vi "Write Target-FIFO 16ch.vi"(0 "16xIQ in":T1=[{"I"=0.0, "Q"=0.0, "overflow"=FALSE}, {"I"=0.0, "Q"=0.0, "overflow"=FALSE}, {"I"=0.0, "Q"=0.0, "overflow"=FALSE}, {"I"=0.0, "Q"=0.0, "overflow"=FALSE}, {"I"=0.0, "Q"=0.0, "overflow"=FALSE}, {"I"=0.0, "Q"=0.0, "overflow"=FALSE}, {"I"=0.0, "Q"=0.0, "overflow"=FALSE}, {"I"=0.0, "Q"=0.0, "overflow"=FALSE}, {"I"=0.0, "Q"=0.0, "overflow"=FALSE}, {"I"=0.0, "Q"=0.0, "overflow"=FALSE}, {"I"=0.0, "Q"=0.0, "overflow"=FALSE}, {"I"=0.0, "Q"=0.0, "overflow"=FALSE}, {"I"=0.0, "Q"=0.0, "overflow"=FALSE}, {"I"=0.0, "Q"=0.0, "overflow"=FALSE}, {"I"=0.0, "Q"=0.0, "overflow"=FALSE}, {"I"=0.0, "Q"=0.0, "overflow"=FALSE}], 7 "Ch select":i32, 9 "input valid":bool) -> (3 "DSP Overflow":bool, 10 "Timed Out?":bool)   [LabVIEW 2015, in "DDC_7976R_v1.lvlib"]
uses:
  DDC_7976R_v1.lvlib
  16xIQData.ctl
  <instrlib>/_niInstr/DSP/v1/Shared/Public/IQ Data.ctl
  <instrlib>/_niInstr/DSP/v1/Shared/niInstr DSP v1 Shared.lvlib
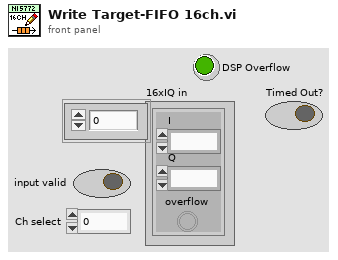
[diagram p1: front panel]
types:
  T1 = typedef "DDC_7976R_v1.lvlib/16xIQData.ctl" = T2[]
  T2 = typedef "niInstr DSP v1 Shared.lvlib/IQ Data.ctl" = cluster{"I":fxp<+/-,18,1>, "Q":fxp<+/-,18,1>, "overflow":bool}
  T3 = typedef "DDC_7976R_v1.lvlib/16xIQData_without_overflow.ctl" = cluster{"I":fxp<+/-,18,1>, "Q":fxp<+/-,18,1>}[]
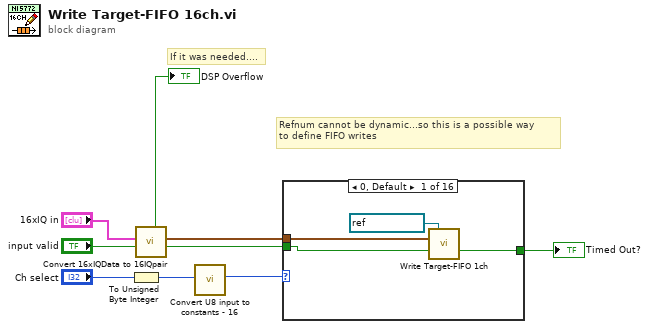
[diagram p0: block diagram]
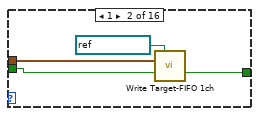
[diagram p2: hidden frame]
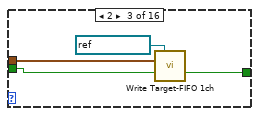
[diagram p3: hidden frame]
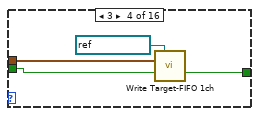
[diagram p4: hidden frame]
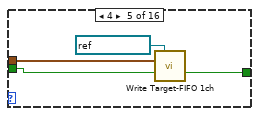
[diagram p5: hidden frame]
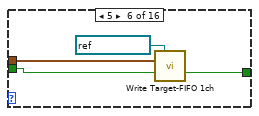
[diagram p6: hidden frame]
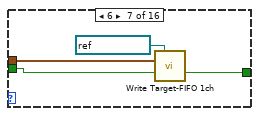
[diagram p7: hidden frame]
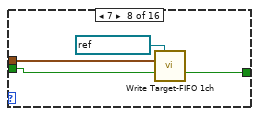
[diagram p8: hidden frame]
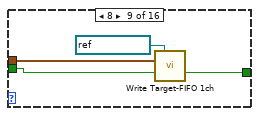
[diagram p9: hidden frame]
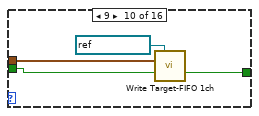
[diagram p10: hidden frame]
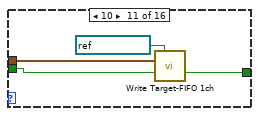
[diagram p11: hidden frame]
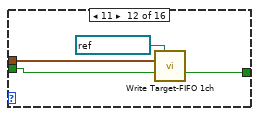
[diagram p12: hidden frame]
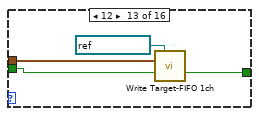
[diagram p13: hidden frame]
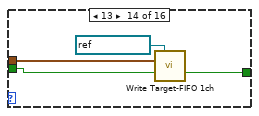
[diagram p14: hidden frame]
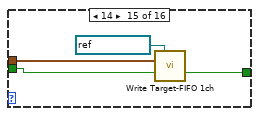
[diagram p15: hidden frame]
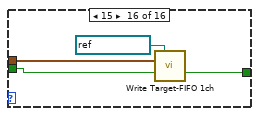
[diagram p16: hidden frame]
diagram:
  # "Refnum cannot be dynamic...so this is a possible way\nto define FIFO writes"
  # "If it was needed...."
  n1 = To Unsigned Byte Integer(number="Ch select") -> (unsigned 8bit integer=w2:u8)
  n2 = call "Convert 16xIQData to 16IQpair.vi"("input valid"="input valid", "16xIQdata in"="16xIQ in") -> ("output valid"=w5:bool, "16xIQpair out"=w6:T3, "Overflow"=→"DSP Overflow":bool)  [unwired: 7 in]
  n3 = call "Convert U8 input to constants - 16.vi"("input U8"=w2) -> ("output U8"=w1:u8)  [unwired: 10 in]
  n4 = case shown="0, Default" w1 {
    tunnel: w6 -> [w13 w17 w21 w25 w29 w33 w37 w41 w45 w49 w53 w57 w61 w65 w69 w73]
    tunnel: w5 -> [w11 w15 w19 w23 w27 w31 w35 w39 w43 w47 w51 w55 w59 w63 w67 w71]
    tunnel: [w10 w14 w18 w22 w26 w30 w34 w38 w42 w46 w50 w54 w58 w62 w66 w70] -> w4
    frame 0, Default {
      n5 = call "Write Target-FIFO 1ch.vi"("FIFO In"=refnum<k21> "FIFO-000", "16IQ in"=w13, "input valid"=w11) -> ("Timed Out?"=w10:bool)  [unwired: 12 in]
    }
    frame 1 {
      n6 = call "Write Target-FIFO 1ch.vi"("FIFO In"=refnum<k21> "FIFO-001", "16IQ in"=w17, "input valid"=w15) -> ("Timed Out?"=w14:bool)  [unwired: 12 in]
    }
    frame 2 {
      n7 = call "Write Target-FIFO 1ch.vi"("FIFO In"=refnum<k21> "FIFO-002", "16IQ in"=w21, "input valid"=w19) -> ("Timed Out?"=w18:bool)  [unwired: 12 in]
    }
    frame 3 {
      n8 = call "Write Target-FIFO 1ch.vi"("FIFO In"=refnum<k21> "FIFO-003", "16IQ in"=w25, "input valid"=w23) -> ("Timed Out?"=w22:bool)  [unwired: 12 in]
    }
    frame 4 {
      n9 = call "Write Target-FIFO 1ch.vi"("FIFO In"=refnum<k21> "FIFO-004", "16IQ in"=w29, "input valid"=w27) -> ("Timed Out?"=w26:bool)  [unwired: 12 in]
    }
    frame 5 {
      n10 = call "Write Target-FIFO 1ch.vi"("FIFO In"=refnum<k21> "FIFO-005", "16IQ in"=w33, "input valid"=w31) -> ("Timed Out?"=w30:bool)  [unwired: 12 in]
    }
    frame 6 {
      n11 = call "Write Target-FIFO 1ch.vi"("FIFO In"=refnum<k21> "FIFO-006", "16IQ in"=w37, "input valid"=w35) -> ("Timed Out?"=w34:bool)  [unwired: 12 in]
    }
    frame 7 {
      n12 = call "Write Target-FIFO 1ch.vi"("FIFO In"=refnum<k21> "FIFO-007", "16IQ in"=w41, "input valid"=w39) -> ("Timed Out?"=w38:bool)  [unwired: 12 in]
    }
    frame 8 {
      n13 = call "Write Target-FIFO 1ch.vi"("FIFO In"=refnum<k21> "FIFO-008", "16IQ in"=w45, "input valid"=w43) -> ("Timed Out?"=w42:bool)  [unwired: 12 in]
    }
    frame 9 {
      n14 = call "Write Target-FIFO 1ch.vi"("FIFO In"=refnum<k21> "FIFO-009", "16IQ in"=w49, "input valid"=w47) -> ("Timed Out?"=w46:bool)  [unwired: 12 in]
    }
    frame 10 {
      n15 = call "Write Target-FIFO 1ch.vi"("FIFO In"=refnum<k21> "FIFO-010", "16IQ in"=w53, "input valid"=w51) -> ("Timed Out?"=w50:bool)  [unwired: 12 in]
    }
    frame 11 {
      n16 = call "Write Target-FIFO 1ch.vi"("FIFO In"=refnum<k21> "FIFO-011", "16IQ in"=w57, "input valid"=w55) -> ("Timed Out?"=w54:bool)  [unwired: 12 in]
    }
    frame 12 {
      n17 = call "Write Target-FIFO 1ch.vi"("FIFO In"=refnum<k21> "FIFO-012", "16IQ in"=w61, "input valid"=w59) -> ("Timed Out?"=w58:bool)  [unwired: 12 in]
    }
    frame 13 {
      n18 = call "Write Target-FIFO 1ch.vi"("FIFO In"=refnum<k21> "FIFO-013", "16IQ in"=w65, "input valid"=w63) -> ("Timed Out?"=w62:bool)  [unwired: 12 in]
    }
    frame 14 {
      n19 = call "Write Target-FIFO 1ch.vi"("FIFO In"=refnum<k21> "FIFO-014", "16IQ in"=w69, "input valid"=w67) -> ("Timed Out?"=w66:bool)  [unwired: 12 in]
    }
    frame 15 {
      n20 = call "Write Target-FIFO 1ch.vi"("FIFO In"=refnum<k21> "FIFO-015", "16IQ in"=w73, "input valid"=w71) -> ("Timed Out?"=w70:bool)  [unwired: 12 in]
    }
  }
  "Timed Out?" <- w4
